vi "Intan_filter_signals_for_display.vi"(1 "Center Traces":bool, 2 "input filter cluster":T1={"LP Filter On/Off"=FALSE, "LP Cutoff (Hz)"=0.0, "HP Filter On/Off"=FALSE, "HP Cutoff (Hz)"=0.0, "Bandstop On/Off"=FALSE, "fl Cutoff (Hz)"=48.0, "fh Cutoff (Hz) "=52.0}, 3 "Sample Rate (Hz)":dbl, 4 "Nchan Array In [Nchans x Nsamps]":i32[][](array[numeric])=array32x200[6400 elements]) -> (0 "Display Signals Out [Nchans x Nsamps]":dbl[][](array[numeric]))   [LabVIEW 2011]
uses:
  <vilib>/Analysis/3filter.llb/Filter Passband Type.ctl
  <vilib>/Analysis/3filter.llb/IIR Cascade Filter with I.C. (DBL).vi
  <vilib>/Analysis/NI_AALBase.lvlib
panel:
  out "iter":i32
  out "Forloopiters":i32
  out "Nsamps":i32
  out "Nchans":i32
  out "chandata":i32[](array[numeric])
  out "filt signal avg":dbl[](array[numeric])
  out "raw signal avg":dbl[](array[numeric])
  out "element subtracted":dbl
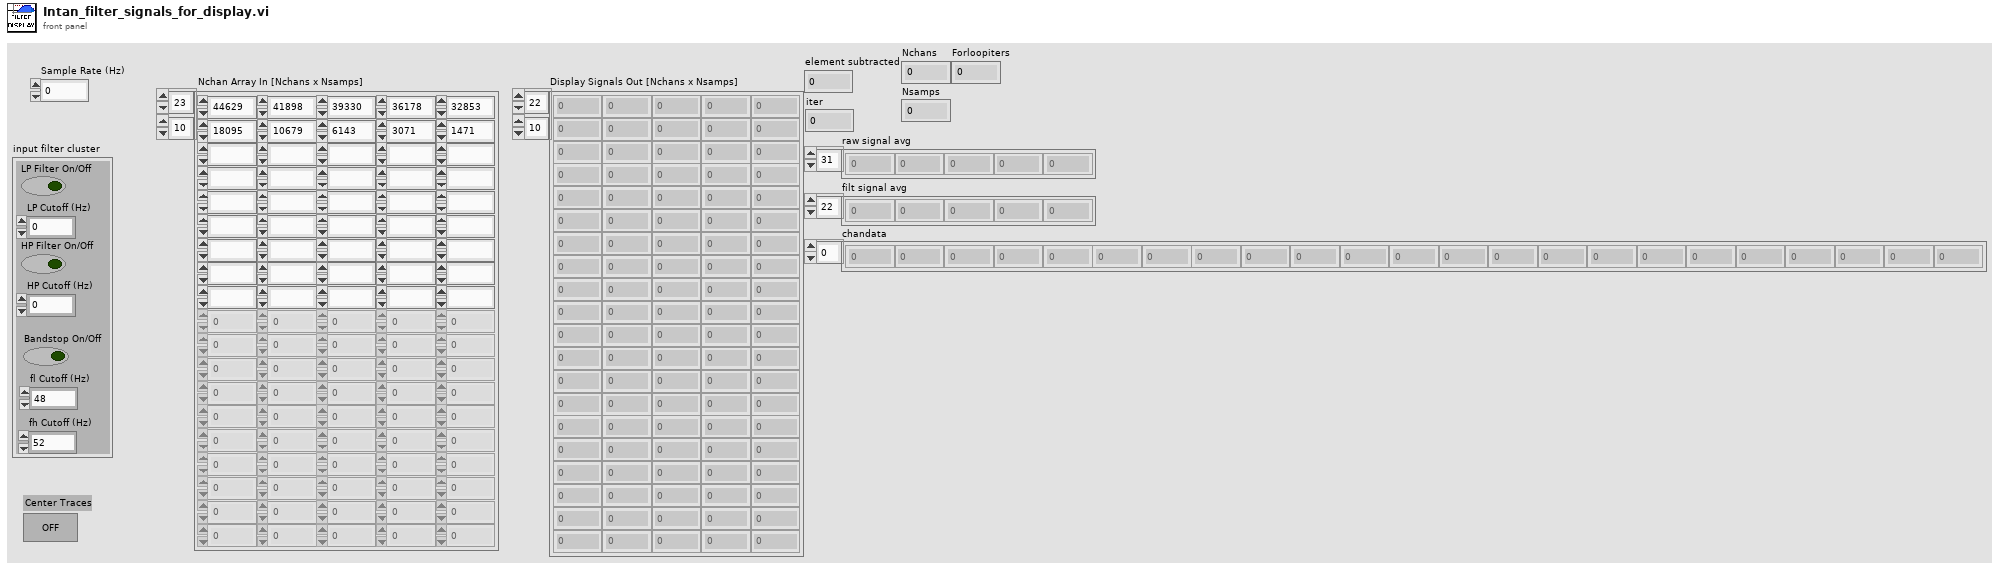
[diagram p1: front panel]
types:
  T1 = cluster{"LP Filter On/Off":bool, "LP Cutoff (Hz)":dbl, "HP Filter On/Off":bool, "HP Cutoff (Hz)":dbl, "Bandstop On/Off":bool, "fl Cutoff (Hz)":dbl, "fh Cutoff (Hz) ":dbl}
  T2 = typedef "NI_AALBase.lvlib/Filter Passband Type.ctl" = enum32{"Lowpass", "Highpass", "Bandpass", "Bandstop"}
  T3 = enum32{"Lowpass", "Highpass", "Bandpass", "Bandstop"}
  T4 = cluster{"filter structure":enum32{"IIR 2nd Order", "IIR 4th Order"}, "Reverse Coefficients":dbl[], "Forward Coefficients":dbl[]}
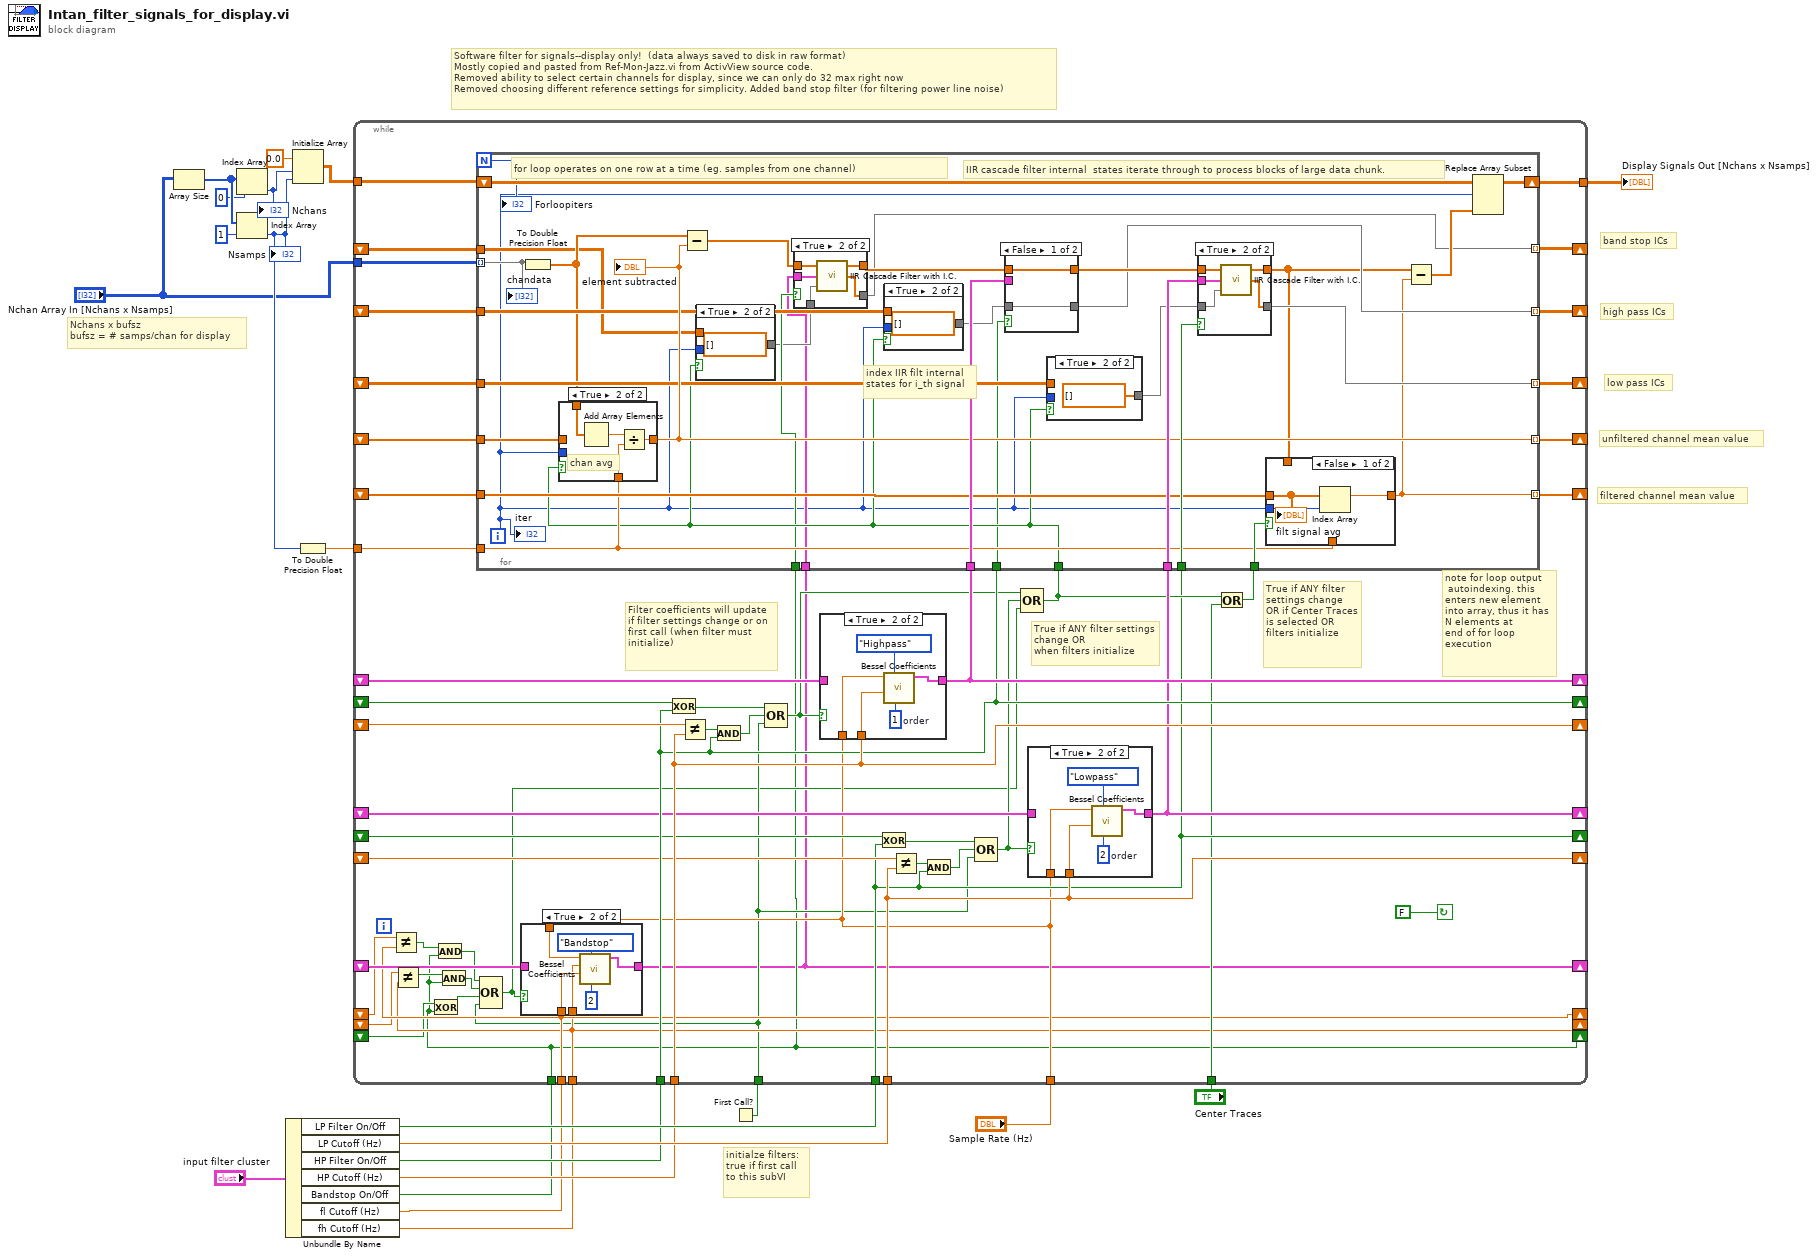
[diagram p0: block diagram]
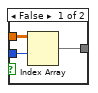
[diagram p5: hidden frame]
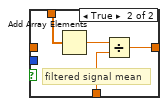
[diagram p7: hidden frame]
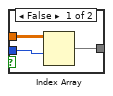
[diagram p8: hidden frame]
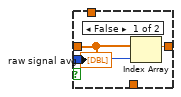
[diagram p9: hidden frame]
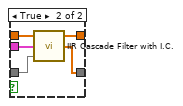
[diagram p11: hidden frame]
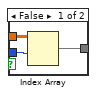
[diagram p12: hidden frame]
diagram:
  # "filtered channel mean value"
  # "unfiltered channel mean value"
  # "low pass ICs"
  # "high pass ICs"
  # "band stop ICs"
  # "Nchans x bufsz \nbufsz = # samps/chan for display"
  # "Software filter for signals--display only!  (data always saved to disk in raw format)\nMostly copied and pasted from Ref-Mon-Jazz.vi from ActivView source code.\nRemoved ability to select certain channels for display, since we can only do 32 max right now\nRemoved choosing different reference settings for simplicity. Added band stop filter (for filtering power line noise)"
  # "initialze filters:\ntrue if first call\nto this subVI"
  n1 = Array Size(array="Nchan Array In [Nchans x Nsamps]") -> (size(s)=w14:i32[])
  n2 = Index Array(array=w14, index=0) -> (element=w11:i32)
  "Nchans" <- w11
  n3 = Index Array(array=w14, index=1) -> (element=w10:i32)
  "Nsamps" <- w10
  n4 = Unbundle By Name("input filter cluster") -> ("LP Filter On/Off"=w21:bool, "LP Cutoff (Hz)"=w19:dbl, "HP Filter On/Off"=w18:bool, "HP Cutoff (Hz)"=w17:dbl, "Bandstop On/Off"=w1:bool, "fl Cutoff (Hz)"=w3:dbl, "fh Cutoff (Hz)"=w2:dbl)
  n5 = Initialize Array(0.0 ("element"), w11, w10) -> (w15:dbl[][])
  n6 = To Double Precision Float(number=w10) -> (double precision float=w9:dbl)
  n7 = First Call?() -> (First Call?: T/F=w7:bool)
  n8 = while {
    shift-left: _ -> [w75]
    shift-right: [w74] -> _
    shift-right: [w67] -> _
    shift-left: _ -> [w68]
    shift-right: [w72] -> _
    shift-left: _ -> [w71]
    shift-right: [w69] -> _
    shift-left: _ -> [w70]
    tunnel: "Nchan Array In [Nchans x Nsamps]" -> [w66]
    tunnel: w9 -> [w65]
    shift-right: [w60] -> _
    shift-left: _ -> [w61]
    shift-right: [w56] -> _
    shift-left: _ -> [w59]
    shift-right: [w57] -> _
    shift-left: _ -> [w58]
    tunnel: w17 -> [w57]
    tunnel: w7 -> [w31]
    tunnel: "Sample Rate (Hz)" -> [w39]
    tunnel: w18 -> [w56]
    shift-right: [w51] -> _
    shift-left: _ -> [w52]
    shift-right: [w45] -> _
    shift-left: _ -> [w50]
    shift-right: [w48] -> _
    shift-left: _ -> [w49]
    tunnel: w19 -> [w48]
    tunnel: w21 -> [w45]
    tunnel: "Center Traces" -> [w42]
    tunnel: w15 -> [w41]
    tunnel: [w40] -> w4
    tunnel: w3 -> [w37]
    tunnel: w2 -> [w35]
    tunnel: w1 -> [w25]
    shift-right: [w24] -> _
    shift-left: _ -> [w38]
    shift-right: [w35] -> _
    shift-left: _ -> [w34]
    shift-right: [w37] -> _
    shift-left: _ -> [w36]
    shift-right: [w25] -> _
    shift-left: _ -> [w33]
    shift-right: [w23] -> _
    shift-left: _ -> [w22]
    stop <- FALSE continue-if-true
    # "note for loop output\n autoindexing. this\nenters new element \ninto array, thus it has\nN elements at \nend of for loop\nexecution"
    # "True if ANY filter settings change\nOR if Center Traces is selected OR filters initialize"
    # "True if ANY filter settings change OR\nwhen filters initialize"
    # "Filter coefficients will update if filter settings change or on first call (when filter must initialize)"
    n9 = Not Equal?(x=w36, y=w37) -> (x != y?=w28:bool)
    n10 = Not Equal?(x=w34, y=w35) -> (x != y?=w27:bool)
    n11 = Exclusive Or(1:w25, 2:w33) -> (0:w32:bool)
    n12 = And(x=w28, y=w25) -> (x .and. y?=w29:bool)
    n13 = And(x=w27, y=w25) -> (x .and. y?=w30:bool)
    n14 = Compound Arithmetic op=OR(w29, w30, w32, w31) -> (w26:bool)
    n15 = case shown="True" w26 {
      tunnel: w37 -> [_ w80]
      tunnel: w35 -> [_ w79]
      tunnel: w39 -> [_ w78]
      tunnel: [w76 w77] -> w24
      tunnel: w38 -> [w76 _]
      frame False {
      }
      frame True {
        n16 = call <vilib>:"Bessel Coefficients.vi"("order"=2, "filter type"=Filter_Passband_Type."Bandstop", "low cutoff freq: fl"=w80, "high cutoff freq: fh"=w79, "sampling freq: fs"=w78) -> ("IIR Filter Cluster"=w77:T4)  [unwired: 5 in, 1 out]
      }
    }
    n17 = Exclusive Or(1:w56, 2:w59) -> (0:w64:bool)
    n18 = Not Equal?(x=w58, y=w57) -> (x != y?=w63:bool)
    n19 = And(x=w63, y=w56) -> (x .and. y?=w62:bool)
    n20 = Compound Arithmetic op=OR(w64, w62, w31) -> (w43:bool)
    n21 = case shown="True" w43 {
      tunnel: w57 -> [_ w93]
      tunnel: w39 -> [_ w92]
      tunnel: [w89 w94] -> w60
      tunnel: w61 -> [w89 _]
      frame False {
      }
      frame True {
        w91 = 1  # order
        n22 = call <vilib>:"Bessel Coefficients.vi"("order"=w91, "filter type"=T3."Highpass", "low cutoff freq: fl"=w93, "sampling freq: fs"=w92) -> ("IIR Filter Cluster"=w94:T4)  [unwired: 6 in, 1 out]
      }
    }
    n23 = Exclusive Or(1:w45, 2:w50) -> (0:w55:bool)
    n24 = Not Equal?(x=w49, y=w48) -> (x != y?=w54:bool)
    n25 = And(x=w54, y=w45) -> (x .and. y?=w53:bool)
    n26 = Compound Arithmetic op=OR(w55, w53, w31) -> (w44:bool)
    n27 = Compound Arithmetic op=OR(w43, w44, w26) -> (w46:bool)
    n28 = case shown="True" w44 {
      tunnel: w48 -> [_ w87]
      tunnel: w39 -> [_ w86]
      tunnel: [w83 w88] -> w51
      tunnel: w52 -> [w83 _]
      frame False {
      }
      frame True {
        w85 = 2  # order
        n29 = call <vilib>:"Bessel Coefficients.vi"("order"=w85, "filter type"=T3."Lowpass", "low cutoff freq: fl"=w87, "sampling freq: fs"=w86) -> ("IIR Filter Cluster"=w88:T4)  [unwired: 6 in, 1 out]
      }
    }
    n30 = Or(x=w46, y=w42) -> (x .or. y?=w47:bool)
    n31 = for {
      N -> [w96]
      tunnel: w75 -> [w118]
      tunnel: [w121] -> w74 mode=indexing
      tunnel: w60 -> [w127]
      tunnel: w46 -> [w105]
      tunnel: w56 -> [w102]
      tunnel: [w124] -> w72 mode=indexing
      tunnel: w71 -> [w117]
      tunnel: w51 -> [w123]
      tunnel: w45 -> [w122]
      tunnel: w70 -> [w113]
      tunnel: [w112] -> w69 mode=indexing
      tunnel: w47 -> [w115]
      tunnel: w68 -> [w120]
      tunnel: [w119] -> w67 mode=indexing
      tunnel: w66 -> [w106] mode=indexing
      tunnel: w65 -> [w108]
      shift-right: [w109] -> w40
      shift-left: w41 -> [w111]
      tunnel: w25 -> [w101]
      tunnel: w24 -> [w99]
      tunnel: [w98] -> w23 mode=indexing
      tunnel: w22 -> [w97]
      i -> [w95]
      # "index IIR filt internal states for i_th signal"
      # "IIR cascade filter internal  states iterate through to process blocks of large data chunk."
      # "for loop operates on one row at a time (eg. samples from one channel)"
      n32 = To Double Precision Float(number=w106) -> (double precision float=w107:dbl[])
      n33 = case shown="True" w105 {
        tunnel: w107 -> [_ w155]
        tunnel: [w150 w154] -> w119
        tunnel: w120 -> [w152 _]
        tunnel: w95 -> [w151 _]
        tunnel: w108 -> [_ w153]
        frame False {
          n34 = Index Array(array=w152, index=w151) -> (element=w150:dbl)
          "raw signal avg" <- w152
        }
        frame True {
          # "chan avg"
          n35 = Add Array Elements(numeric array=w155) -> (sum=w156:dbl)
          n36 = Divide(x=w156, y=w153) -> (x/y=w154:dbl)
        }
      }
      "element subtracted" <- w119
      n37 = Subtract(x=w107, y=w119) -> (x-y=w103:dbl[])
      n38 = case shown="True" w105 {
        tunnel: [w128 dbl[] [] ("Initial Filter State")] -> w100
        tunnel: w97 -> [w130 _]
        tunnel: w95 -> [w129 _]
        frame False {
          n39 = Index Array(array=w130, index (row)=w129) -> (element=w128:dbl[])  [unwired: 1 in]
        }
        frame True {
        }
      }
      n40 = case shown="True" w101 {
        tunnel: [w132 w138] -> w98
        tunnel: [w133 w137] -> w104
        tunnel: w103 -> [w133 w136]
        tunnel: w100 -> [w132 w135]
        tunnel: w99 -> [_ w134]
        frame False {
        }
        frame True {
          n41 = call-poly <vilib>:"IIR Cascade Filter with I.C..vi"("Initial Filter State"=w135, "IIR Filter Cluster"=w134, "X"=w136) -> ("Final Filter State"=w138:dbl[], "Filtered X"=w137:dbl[])  [unwired: 1 out]
        }
      }
      n42 = case shown="True" w105 {
        tunnel: [w171 dbl[] [] ("Initial Filter State")] -> w126
        tunnel: w118 -> [w173 _]
        tunnel: w95 -> [w172 _]
        frame False {
          n43 = Index Array(array=w173, index (row)=w172) -> (element=w171:dbl[])  [unwired: 1 in]
        }
        frame True {
        }
      }
      n44 = case shown="False" w102 {
        tunnel: w127 -> [_ w170]
        tunnel: [w164 w169] -> w121
        tunnel: w126 -> [w164 w168]
        tunnel: [w165 w167] -> w125
        tunnel: w104 -> [w165 w166]
        frame False {
        }
        frame True {
          n45 = call-poly <vilib>:"IIR Cascade Filter with I.C..vi"("Initial Filter State"=w168, "IIR Filter Cluster"=w170, "X"=w166) -> ("Final Filter State"=w169:dbl[], "Filtered X"=w167:dbl[])  [unwired: 1 out]
        }
      }
      n46 = case shown="True" w105 {
        tunnel: [w146 dbl[] [] ("Initial Filter State")] -> w116
        tunnel: w117 -> [w148 _]
        tunnel: w95 -> [w147 _]
        frame False {
          n47 = Index Array(array=w148, index (row)=w147) -> (element=w146:dbl[])  [unwired: 1 in]
        }
        frame True {
        }
      }
      n48 = case shown="True" w122 {
        tunnel: w123 -> [_ w163]
        tunnel: [w157 w162] -> w124
        tunnel: w116 -> [w157 w161]
        tunnel: [w158 w160] -> w114
        tunnel: w125 -> [w158 w159]
        frame False {
        }
        frame True {
          n49 = call-poly <vilib>:"IIR Cascade Filter with I.C..vi"("Initial Filter State"=w161, "IIR Filter Cluster"=w163, "X"=w159) -> ("Final Filter State"=w162:dbl[], "Filtered X"=w160:dbl[])  [unwired: 1 out]
        }
      }
      n50 = case shown="False" w115 {
        tunnel: w114 -> [_ w143]
        tunnel: [w139 w145] -> w112
        tunnel: w113 -> [w141 _]
        tunnel: w95 -> [w140 _]
        tunnel: w108 -> [_ w142]
        frame False {
          n51 = Index Array(array=w141, index=w140) -> (element=w139:dbl)
          "filt signal avg" <- w141
        }
        frame True {
          # "filtered signal mean"
          n52 = Add Array Elements(numeric array=w143) -> (sum=w144:dbl)
          n53 = Divide(x=w144, y=w142) -> (x/y=w145:dbl)
        }
      }
      n54 = Subtract(x=w114, y=w112) -> (x-y=w110:dbl[])
      n55 = Replace Array Subset(array=w111, new element=w110, index (row)=w95) -> (w109:dbl[][])  [unwired: 1 in]
      "chandata" <- w106
      "Forloopiters" <- w96
      "iter" <- w95
    }
  }
  "Display Signals Out [Nchans x Nsamps]" <- w4
